vi "Rabi Pulse 2.vi"() -> ()   [LabVIEW 2012]
uses:
  <vilib>/Utility/file.llb/Write To Spreadsheet File (DBL).vi
  <vilib>/DAQmx/create/channels.llb/DAQmx Create Channel (DI-Digital Input).vi
  <vilib>/DAQmx/read.llb/DAQmx Read (Digital Bool 1Line 1Point).vi
panel:
  out "Run":bool
  out "size(s)":i32=225
  in  "file path (dialog if empty)":path=path "C:/Users/Ouyang Group/Documents/Data/12-5-13/Rabi pulse sequence 7"
  in  "AOM Pulse length":dbl=3e-07
  in  "N Loop":i32=25000
  in  "Path to spinapi.dll":path=path "C:/SpinCore/SpinAPI/dll/spinapi64.dll"
  in  "stop":bool
  in  "start/restart":bool
  in  "MW width Max":dbl=5e-07
  in  "MW width step size":dbl=2e-09
  in  "MW width Min":dbl=5e-08
  in  "clock_freq (MHz)":dbl=300.0
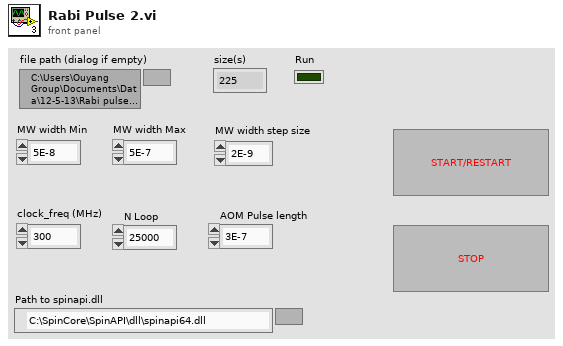
[diagram p1: front panel]
types:
  T1 = cluster{"Instruct Data":i32, "Op Code":i32, "Flags":bool[], "Comments":string, "Time (s)":dbl}
  T2 = enum16{"Pulse Program", "Frequency Registers", "TX Phase Registers", "RX Phase Registers"}
  T3 = cluster{"Instruct Data":i32, "Op Code":i32, "Flags":bool[], "Comments":string, "Time (s)":dbl}[]
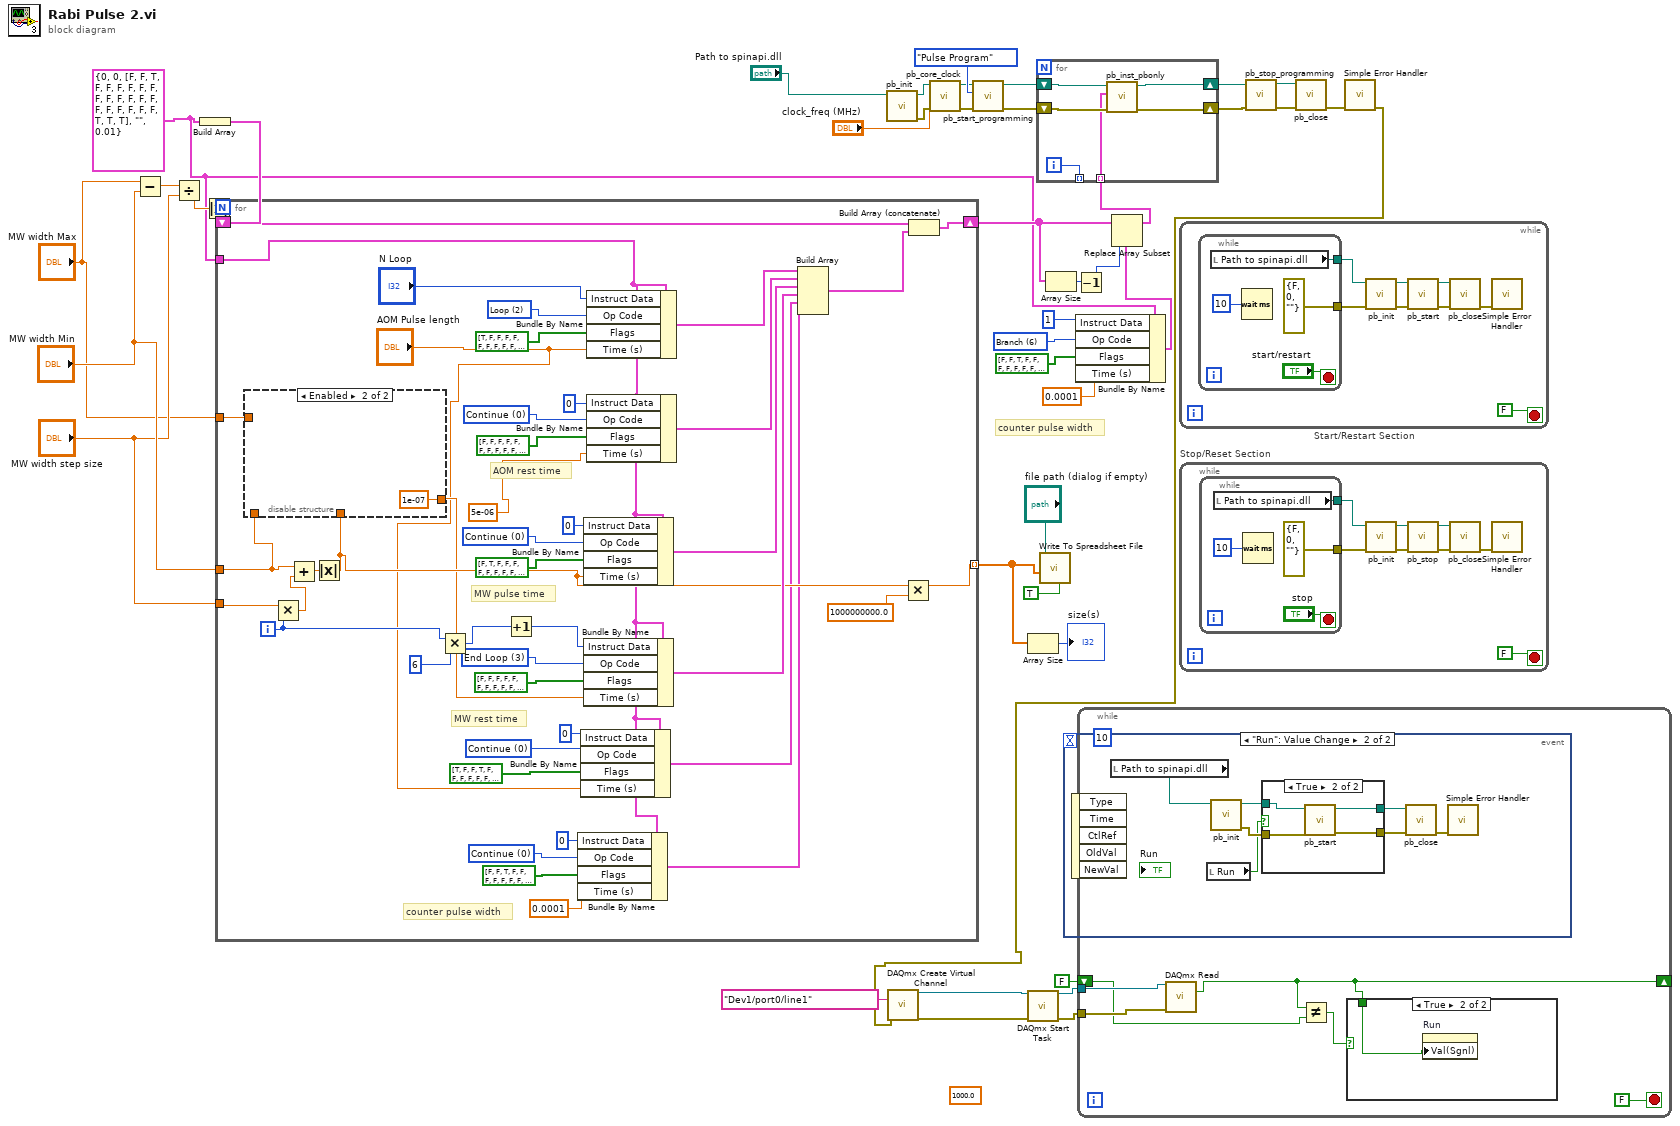
[diagram p0: block diagram]
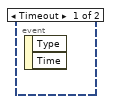
[diagram p2: hidden frame]
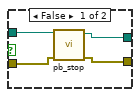
[diagram p3: hidden frame]
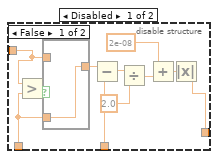
[diagram p5: hidden frame]
diagram:
  w5 = 6 items=["Continue", "Stop", "Loop", "End Loop", "JSR", "RTS", "Branch", "Long Delay", "Wait"] ("Op Code")
  (unwired) 1000.0 ("rate")
  w2 = T1 {"Instruct Data"=0, "Op Code"=0, "Flags"=[FALSE, FALSE, TRUE, FALSE, FALSE, FALSE, FALSE, FALSE, FALSE, FALSE, FALSE, FALSE, FALSE, FALSE, FALSE, FALSE, FALSE, FALSE, FALSE, FALSE, FALSE, TRUE, TRUE, TRUE], "Comments"="", "Time (s)"=0.01} ("PB Inst 2")
  # "counter pulse width"
  n1 = Subtract(x="MW width Max", y="MW width Min") -> (x-y=w30:dbl)
  n2 = Divide(x=w30, y="MW width step size") -> (x/y=w29:dbl)
  n3 = Build Array(w2) -> (w26:T3)
  n4 = Absolute Value(x=w29) -> (abs(x)=w11:dbl)
  n5 = for {
    N: w11 -> [_]
    tunnel: "MW width Min" -> [w52]
    tunnel: "MW width step size" -> [w85]
    tunnel: [w57] -> w21 mode=indexing
    tunnel: w2 -> [w49]
    shift-right: [w82] -> w10
    shift-left: w26 -> [w83]
    tunnel: "MW width Max" -> [w53]
    i -> [w58]
    w46 = 0 items=["Continue", "Stop", "Loop", "End Loop", "JSR", "RTS", "Branch", "Long Delay", "Wait"] ("Op Code")
    w70 = 0 items=["Continue", "Stop", "Loop", "End Loop", "JSR", "RTS", "Branch", "Long Delay", "Wait"] ("Op Code")
    w72 = 3 items=["Continue", "Stop", "Loop", "End Loop", "JSR", "RTS", "Branch", "Long Delay", "Wait"] ("Op Code")
    w75 = 0 items=["Continue", "Stop", "Loop", "End Loop", "JSR", "RTS", "Branch", "Long Delay", "Wait"] ("Op Code")
    w78 = 0 items=["Continue", "Stop", "Loop", "End Loop", "JSR", "RTS", "Branch", "Long Delay", "Wait"] ("Op Code")
    w80 = 2 items=["Continue", "Stop", "Loop", "End Loop", "JSR", "RTS", "Branch", "Long Delay", "Wait"] ("Op Code")
    # "counter pulse width"
    # "MW rest time"
    # "MW pulse time"
    # "AOM rest time"
    n6 = Multiply(x=w85, y=w58) -> (x*y=w84:dbl)
    n7 = Add(x=w52, y=w84) -> (x+y=w55:dbl)
    n8 = Absolute Value(x=w55) -> (abs(x)=w54:dbl)
    n9 = disable-structure shown="Enabled" {
      disable-tunnel: [w91 1e-07] -> w51
      disable-tunnel: w54 -> [w90 _]
      disable-tunnel: w53 -> [w87 _]
      disable-tunnel: w52 -> [w86 _]
      frame Disabled {
        n10 = Greater?(x=w87, y=w86) -> (0:w89:bool)
        n11 = case shown="False" w89 {
          tunnel: [w97 w98] -> w88
          tunnel: w87 -> [_ w98]
          tunnel: w86 -> [w97 _]
          frame False {
          }
          frame True {
          }
        }
        n12 = Subtract(x=w88, y=w90) -> (x-y=w96:dbl)
        n13 = Divide(x=w96, y=2.0) -> (x/y=w94:dbl)
        n14 = Add(x=2e-08, y=w94) -> (x+y=w92:dbl)
        n15 = Absolute Value(x=w92) -> (abs(x)=w91:dbl)
      }
      frame Enabled {
      }
    }
    n16 = Multiply(x=w58, y=6) -> (x*y=w59:i32)
    n17 = Increment(x=w59) -> (x+1=w61:i32)
    n18 = Bundle By Name(cluster=w49, "Instruct Data"=0, "Op Code"=w70, "Flags"=bool[] [FALSE, FALSE, TRUE, FALSE, FALSE, FALSE, FALSE, FALSE, FALSE, FALSE, FALSE, FALSE, FALSE, FALSE, FALSE, FALSE, FALSE, FALSE, FALSE, FALSE, FALSE, TRUE, TRUE, TRUE], "Time (s)"=0.0001) -> (w50:T1)
    n19 = Bundle By Name(cluster=w49, "Instruct Data"=0, "Op Code"=w46, "Flags"=bool[] [TRUE, FALSE, FALSE, TRUE, FALSE, FALSE, FALSE, FALSE, FALSE, FALSE, FALSE, FALSE, FALSE, FALSE, FALSE, FALSE, FALSE, FALSE, FALSE, FALSE, FALSE, TRUE, TRUE, TRUE], "Time (s)"="AOM Pulse length") -> (w48:T1)
    n20 = Bundle By Name(cluster=w49, "Instruct Data"=0, "Op Code"=w75, "Flags"=bool[] [FALSE, TRUE, FALSE, FALSE, FALSE, FALSE, FALSE, FALSE, FALSE, FALSE, FALSE, FALSE, FALSE, FALSE, FALSE, FALSE, FALSE, FALSE, FALSE, FALSE, FALSE, TRUE, TRUE, TRUE], "Time (s)"=w54) -> (w65:T1)
    n21 = Bundle By Name(cluster=w49, "Instruct Data"=w61, "Op Code"=w72, "Flags"=bool[] [FALSE, FALSE, FALSE, FALSE, FALSE, FALSE, FALSE, FALSE, FALSE, FALSE, FALSE, FALSE, FALSE, FALSE, FALSE, FALSE, FALSE, FALSE, FALSE, FALSE, FALSE, TRUE, TRUE, TRUE], "Time (s)"=w51) -> (w64:T1)
    n22 = Bundle By Name(cluster=w49, "Instruct Data"="N Loop", "Op Code"=w80, "Flags"=bool[] [TRUE, FALSE, FALSE, FALSE, FALSE, FALSE, FALSE, FALSE, FALSE, FALSE, FALSE, FALSE, FALSE, FALSE, FALSE, FALSE, FALSE, FALSE, FALSE, FALSE, FALSE, TRUE, TRUE, TRUE], "Time (s)"="AOM Pulse length") -> (w67:T1)
    n23 = Bundle By Name(cluster=w49, "Instruct Data"=0, "Op Code"=w78, "Flags"=bool[] [FALSE, FALSE, FALSE, FALSE, FALSE, FALSE, FALSE, FALSE, FALSE, FALSE, FALSE, FALSE, FALSE, FALSE, FALSE, FALSE, FALSE, FALSE, FALSE, FALSE, FALSE, TRUE, TRUE, TRUE], "Time (s)"=5e-06) -> (w66:T1)
    n24 = Build Array(w67, w66, w65, w64, w48, w50) -> (w60:T3)
    n25 = Multiply(x=w54, y=1000000000.0) -> (x*y=w57:dbl)
    n26 = Build Array (concatenate)(w83, w60) -> (w82:T3)
  }
  n27 = call "pb_init.vi"("path in"="Path to spinapi.dll") -> ("error out"=w37:errorcluster, "path out"=w39:path)  [unwired: 3 in, 6 out]
  n28 = call "pb_core_clock.vi"("error in (no error)"=w37, "clock_freq (MHz)"="clock_freq (MHz)", "path in"=w39) -> ("error out"=w36:errorcluster, "path out"=w38:path)  [unwired: 7 in]
  n29 = call "pb_start_programming.vi"("error in (no error)"=w36, "Device"=T2."Pulse Program", "path in"=w38) -> ("error out"=w33:errorcluster, "path out"=w34:path)  [unwired: 1 in, 6 out]
  n30 = Array Size(array=w21) -> (size(s)=→"size(s)":i32)
  n31 = call-poly <vilib>:"Write To Spreadsheet File.vi"("transpose? (no:F)"=TRUE, "1D data"=w21, "file path (dialog if empty)"="file path (dialog if empty)") -> ()  [unwired: 5 in, 1 out]
  n32 = Array Size(array=w10) -> (size(s)=w9:i32)
  n33 = event shown="[1] \"Run\": Value Change" {
    selector: _ -> [_ _]
    dyn-events: _ -> [_ _]
    timeout: _ -> [_ _]
    event Timeout {
      n34 = event-data() -> ()  [unwired: 1 in, 2 out]
    }
    event "Run": Value Change {
      n35 = event-data() -> ()  [unwired: 1 in, 5 out]
      n36 = local read "Path to spinapi.dll"() -> (w100:path)
      n37 = local read "Run"() -> (w104:bool)
      n38 = call "pb_init.vi"("path in"=w100) -> ("error out"=w105:errorcluster, "path out"=w106:path)  [unwired: 2 in, 7 out]
      n39 = case shown="True" w104 {
        tunnel: w106 -> [w110 w114]
        tunnel: w105 -> [w109 w113]
        tunnel: [w108 w112] -> w102
        tunnel: [w107 w111] -> w101
        frame False {
          n40 = call "pb_stop.vi"("error in (no error)"=w109, "path in"=w110) -> ("error out"=w107:errorcluster, "path out"=w108:path)  [unwired: 8 out]
        }
        frame True {
          n41 = call "pb_start.vi"("error in (no error)"=w113, "path in"=w114) -> ("error out"=w111:errorcluster, "path out"=w112:path)  [unwired: 1 in, 7 out]
        }
      }
      n42 = call "pb_close.vi"("error in (no error)"=w101, "path in"=w102) -> ("error out"=w103:errorcluster)  [unwired: 9 out]
      n43 = call <vilib>:"Simple Error Handler.vi"("error in (no error)"=w103) -> ()  [unwired: 1 in, 8 out]
    }
  }
  n44 = Decrement(x=w9) -> (x-1=w8:i32)
  n45 = Bundle By Name(cluster=w2, "Instruct Data"=1, "Op Code"=w5, "Flags"=bool[] [FALSE, FALSE, TRUE, FALSE, FALSE, FALSE, FALSE, FALSE, FALSE, FALSE, FALSE, FALSE, FALSE, FALSE, FALSE, FALSE, FALSE, FALSE, FALSE, FALSE, FALSE, TRUE, TRUE, TRUE], "Time (s)"=0.0001) -> (w3:T1)
  n46 = Replace Array Subset(array=w10, new element=w3, index=w8) -> (w1:T3)
  n47 = for {
    shift-right: [w118] -> w32
    shift-left: w34 -> [w120]
    shift-right: [w117] -> w31
    shift-left: w33 -> [w119]
    tunnel: [w116] -> _ mode=indexing
    tunnel: w1 -> [w115] mode=indexing
    i -> [w116]
    n48 = call "pb_inst_pbonly.vi"("error in (no error)"=w119, "PB Instruction"=w115, "path in"=w120) -> ("error out"=w117:errorcluster, "path out"=w118:path)  [unwired: 2 in, 5 out]
  }
  n49 = while "Start/Restart Section" {
    stop <- FALSE stop-if-true
    n50 = while {
      tunnel: [errorcluster {"status"=FALSE, "code"=0, "source"=""} ("error in (no error)")] -> w125
      tunnel: [w129] -> w121
      stop <- "start/restart" stop-if-true
      n51 = local read "Path to spinapi.dll"() -> (w129:path)
      n52 = Wait (ms)(milliseconds to wait=u32 10) -> ()  [unwired: 1 out]
    }
    n53 = call "pb_init.vi"("error in (no error)"=w125, "path in"=w121) -> ("error out"=w124:errorcluster, "path out"=w127:path)  [unwired: 1 in, 7 out]
    n54 = call "pb_start.vi"("error in (no error)"=w124, "path in"=w127) -> ("error out"=w123:errorcluster, "path out"=w128:path)  [unwired: 1 in, 7 out]
    n55 = call "pb_close.vi"("error in (no error)"=w123, "path in"=w128) -> ("error out"=w122:errorcluster)  [unwired: 9 out]
    n56 = call <vilib>:"Simple Error Handler.vi"("error in (no error)"=w122) -> ()  [unwired: 1 in, 8 out]
  }
  n57 = while "Stop/Reset Section" {
    stop <- FALSE stop-if-true
    n58 = while {
      tunnel: [errorcluster {"status"=FALSE, "code"=0, "source"=""} ("error in (no error)")] -> w137
      tunnel: [w141] -> w133
      stop <- "stop" stop-if-true
      n59 = local read "Path to spinapi.dll"() -> (w141:path)
      n60 = Wait (ms)(milliseconds to wait=u32 10) -> ()  [unwired: 1 out]
    }
    n61 = call "pb_init.vi"("error in (no error)"=w137, "path in"=w133) -> ("error out"=w136:errorcluster, "path out"=w139:path)  [unwired: 1 in, 7 out]
    n62 = call "pb_stop.vi"("error in (no error)"=w136, "path in"=w139) -> ("error out"=w135:errorcluster, "path out"=w140:path)  [unwired: 8 out]
    n63 = call "pb_close.vi"("error in (no error)"=w135, "path in"=w140) -> ("error out"=w134:errorcluster)  [unwired: 9 out]
    n64 = call <vilib>:"Simple Error Handler.vi"("error in (no error)"=w134) -> ()  [unwired: 1 in, 8 out]
  }
  n65 = call "pb_stop_programming.vi"("error in (no error)"=w31, "path in"=w32) -> ("error out"=w40:errorcluster, "path out"=w41:path)  [unwired: 1 in, 7 out]
  n66 = call "pb_close.vi"("error in (no error)"=w40, "path in"=w41) -> ("error out"=w24:errorcluster)  [unwired: 9 out]
  n67 = call <vilib>:"Simple Error Handler.vi"("error in (no error)"=w24) -> ("error out"=w15:errorcluster)  [unwired: 1 in, 7 out]
  n68 = call-poly <vilib>:"DAQmx Create Virtual Channel.vi"("lines"=tag "Dev1/port0/line1", "error in"=w15) -> ("task out"=w13:refnum<k21>, "error out"=w12:errorcluster)  [unwired: 12 in]
  n69 = call <vilib>:"DAQmx Start Task.vi"("task/channels in"=w13, "error in"=w12) -> ("task out"=w14:refnum<k21>, "error out"=w17:errorcluster)  [unwired: 12 in]
  n70 = while {
    tunnel: w14 -> [w151]
    tunnel: w17 -> [w150]
    shift-right: [w147] -> _
    shift-left: FALSE ("data") -> [w149]
    stop <- FALSE stop-if-true
    w145 = 10
    n71 = call-poly <vilib>:"DAQmx Read.vi"("task/channels in"=w151, "error in"=w150) -> ("data"=w147:bool)  [unwired: 11 in, 2 out]
    n72 = Not Equal?(x=w147, y=w149) -> (x != y?=w148:bool)
    n73 = case shown="True" w148 {
      tunnel: w147 -> [_ w152]
      frame False {
      }
      frame True {
        n74 = property on="Run" class="Bool (strict)"("Val(Sgnl)"=w152) -> ()  [unwired: 2 in, 2 out]
      }
    }
  }
